vi "Test Get Debug Log Pause Refreshing.vi"(8 "error in (no error)":errorcluster, 11 "Test Case In":refnum<class "Debugger Test.lvclass">) -> (0 "error out":errorcluster, 3 "Test Case Out":refnum<class "Debugger Test.lvclass">)   [LabVIEW 2020, in "Debugger Test.lvclass"]
uses:
  Debugger Test.lvclass
  C:/Program Files (x86)/National Instruments/LabVIEW 2020/vi.lib/Astemes/LUnit/Test Case.lvclass
  source/Debugger/Debugger.lvclass
  C:/Git/astemes-triarc-debugger/source/Process/Debug Process.lvclass
  source/Debug Data/Raw Debug Data.ctl
  source/Debug Data/Debug Data.lvclass/Debug Data.ctl
  source/Process/Debug Process.lvclass/Debug Process.ctl
  <vilib>/Astemes/LUnit/Test Case.lvclass/Test Case.ctl
  01074fa8-ee8a-411d-bc8b-fc92c4f90959.vi
  <vilib>/AdvancedString/Delimited String to 1D String Array.vi
  source/Process/Public/Lifecycle/Get Lifecycle State.vi
  <vilib>/Astemes/Triarc Framework/Broadcast Event Helpers/Execution timer.vi
  source/Process/Private/SubVIs/Wait for finish.vi
  source/Process/Protected/Messaging/Enqueue Message.vi
  source/Process/Private/SubVIs/Set Lifecycle State.vi
  <vilib>/Astemes/LUnit/Palette/Pass.vi
  <vilib>/Astemes/LUnit/Palette/Fail.vi
  <vilib>/Astemes/LUnit/Compare Variants.vi
  <vilib>/Astemes/LUnit/Describe Comparison.vi
  <vilib>/Astemes/LUnit/Set Assertion Type.vi
  <vilib>/Utility/error.llb/Clear Errors.vi
  <vilib>/Astemes/LUnit/Add test result.vi
  <vilib>/Astemes/LUnit/Variant to string.vi
  <vilib>/Astemes/LUnit/LUnit Record Assertion Result.vi
  <vilib>/Astemes/LUnit/LUnit Aggregate Assertion Results.vi
  <vilib>/Astemes/LUnit/Method Result/LUnit Merge Status.vi
  <vilib>/Astemes/LUnit/LUnit Concatenate result strings.vi
  <vilib>/Utility/error.llb/Error Cluster From Error Code.vi
  <vilib>/Astemes/Triarc Framework/Broadcast Event Helpers/Dequeue Broadcast Message.vi
  <vilib>/Utility/Data Type/Get Type Information.vi
  <vilib>/Utility/LVClass/Get LV Class Name.vi
  source/Debug Data/Debug Data.lvclass
  source/Process/Debug Process.lvclass
  <vilib>/Astemes/Triarc Framework/Broadcast Event Helpers/Broadcast Event Helpers.lvlib
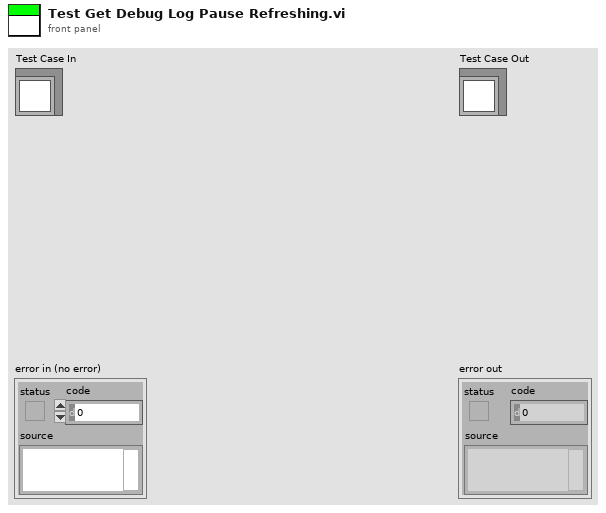
[diagram p1: front panel]
types:
  T1 = typedef "Debug Data.lvclass/Raw Debug Data.ctl" = cluster{"Action":string, "Call Chain":string, "Process":string, "Message":string, "Message Data":variant, "Time":dbl}
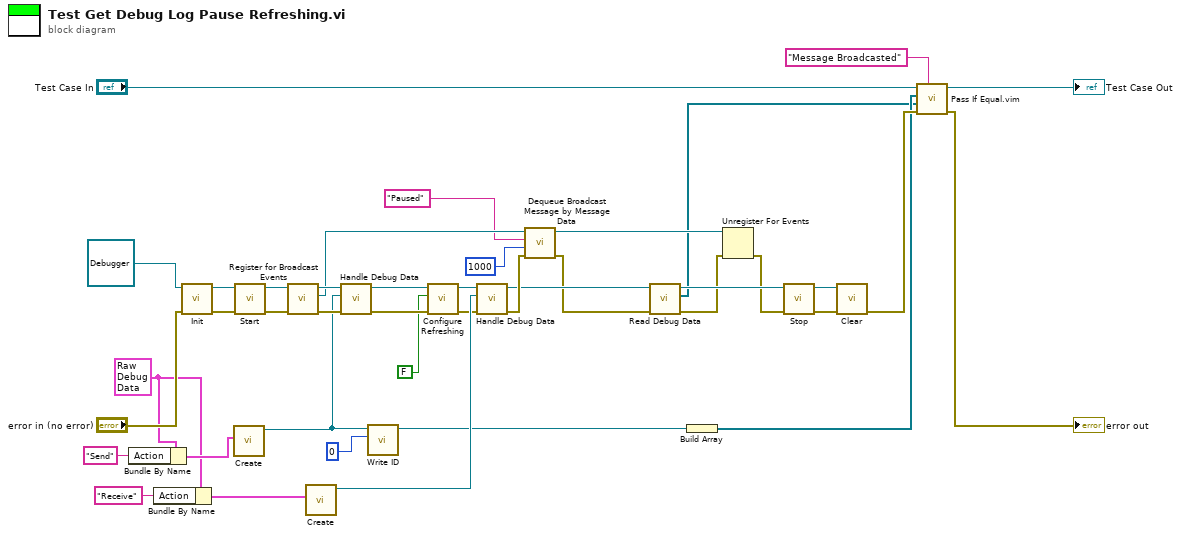
[diagram p0: block diagram]
diagram:
  w18 = T1 {"Action"="", "Call Chain"="", "Process"="", "Message"="", "Message Data"=variant, "Time"=0.0} ("Debug Data Cluster")
  n1 = Bundle By Name(cluster=w18, "Action"="Send" ("Process")) -> (w23:T1)
  n2 = Bundle By Name(cluster=w18, "Action"="Receive" ("Process")) -> (w19:T1)
  n3 = call-dynamic "Init.vi"("error in (no error)"="error in (no error)", "Process In"=refnum<class "Debugger.lvclass"> refnum ("Debug Data Event In 2")) -> ("error out"=w37:errorcluster, "Process Out"=w38:refnum<class "Debugger.lvclass">)  [unwired: 8 in]
  n4 = call "Create.vi"("Debug Data Cluster"=w23) -> ("Debug Data out"=w8:refnum<class "Debug Data.lvclass">)  [unwired: 9 in, 1 out]
  n5 = call "Start.vi"("error in (no error)"=w37, "Process In"=w38) -> ("error out"=w35:errorcluster, "Process Out"=w36:refnum<class "Debugger.lvclass">)  [unwired: 7 in, 1 out]
  n6 = call "Register for Broadcast Events.vi"("error in (no error)"=w35, "Process In"=w36) -> ("error out"=w34:errorcluster, "Event Registration Refnum Out"=w24:refnum<event-registration>, "Process Out"=w30:refnum<class "Debugger.lvclass">)  [unwired: 7 in]
  n7 = call "Create.vi"("Debug Data Cluster"=w19) -> ("Debug Data out"=w10:refnum<class "Debug Data.lvclass">)  [unwired: 9 in, 1 out]
  n8 = call-dynamic "Handle Debug Data.vi"("error in (no error)"=w34, "Debug Data.lvclass"=w8, "Debug Data Event In"=w30) -> ("error out"=w21:errorcluster, "Debug Data Event Out"=w17:refnum<class "Debugger.lvclass">)  [unwired: 7 in]
  n9 = call "Write ID.vi"("ID"=u32 0, "Debug Data in"=w8) -> ("Debug Data out"=w7:refnum<class "Debug Data.lvclass">)  [unwired: 8 in, 1 out]
  n10 = call "Configure Refreshing.vi"("error in (no error)"=w21, "Refresh?"=FALSE ("Show Send?"), "Debugger In"=w17) -> ("error out"=w4:errorcluster, "Debugger Out"=w5:refnum<class "Debugger.lvclass">)  [unwired: 7 in]
  n11 = call-dynamic "Handle Debug Data.vi"("error in (no error)"=w4, "Debug Data.lvclass"=w10, "Debug Data Event In"=w5) -> ("error out"=w3:errorcluster, "Debug Data Event Out"=w2:refnum<class "Debugger.lvclass">)  [unwired: 7 in]
  n12 = call <vilib>:"Dequeue Broadcast Message by Message Data.vi"("error in (no error)"=w3, "Timeout (-1)"=1000, "Message Data"="Paused" ("Message"), "Event Registration Refnum"=w24) -> ("error out"=w1:errorcluster, "Event Registration Refnum Out"=w13:refnum<event-registration>)  [unwired: 3 in, 3 out]
  n13 = call "Read Debug Data.vi"("error in (no error)"=w1, "Debugger In"=w2) -> ("error out"=w16:errorcluster, "Data Log"=w6:refnum<class "Debug Data.lvclass">[], "Debugger Out"=w33:refnum<class "Debugger.lvclass">)  [unwired: 7 in]
  n14 = Build Array(w7) -> (w25:refnum<class "Debug Data.lvclass">[])
  n15 = Unregister For Events(event registration refnum=w13, error in=w16) -> (error out=w15:errorcluster)
  n16 = call "Stop.vi"("error in (no error)"=w15, "Process In"=w33) -> ("error out"=w31:errorcluster, "Process Out"=w32:refnum<class "Debugger.lvclass">)  [unwired: 7 in, 1 out]
  n17 = call-dynamic "Clear.vi"("error in (no error)"=w31, "Process In"=w32) -> ("error out"=w27:errorcluster)  [unwired: 9 in]
  n18 = call "Pass If Equal.vim"("Description"="Message Broadcasted", "error in (no error)"=w27, "Actual"=w6, "Expected"=w25, "LUnit Test Case In"="Test Case In") -> ("error out"=→"error out":errorcluster, "LUnit Test Case Out"=→"Test Case Out":refnum<class "Debugger Test.lvclass">)  [unwired: 5 in]
